vi "PH_VacuumControl.Show Trend.vi"(0 "i ref in":refnum<vi>, 5 "error in":errorcluster) -> (14 "i ref out":refnum<vi>, 19 "error out":errorcluster)   [LabVIEW 2014, in "PH_VacuumControl.lvlib"]
doc: "This VI shows the Trend data."
uses:
  PH_VacuumControl.lvlib
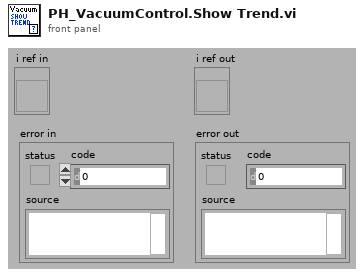
[diagram p1: front panel]
types:
  T1 = typedef "PH_VacuumControl.lvlib/PH_VacuumControl.i attribute.ctl" = cluster{"GUI Refs":cluster{"Exit":refnum<vi>, "Set Unit":refnum<vi>, "Device found":refnum<vi>, "Busy":refnum<vi>, "State":refnum<vi>, "Delete":refnum<vi>, "Channels":refnum<vi>, "Channel Name":refnum<vi>, "Trend":refnum<vi>, "Logarithmic":refnum<vi>, "Limit reached":refnum<vi>, "Channel Name 1 MT":refnum<vi>, "Channel Name 2 MT":refnum<vi>, "Trend MT":refnum<vi>, "Logarithmic MT":refnum<vi>, "Limit reached MT":refnum<vi>}, "Device found":bool, "Busy":bool, "Selected Unit":i32, "Channels [mbar]":T2, "Channel Names":cluster{"Channel 1":string, "Channel 2":string, "Channel 3":string, "Channel 4":string, "Channel 5":string, "Channel 6":string}, "Status":T3, "AGCxxx VISA Cluster":T4, "Instr Firmware Revision":string, "Service IDs Pressure":cluster{"Channel 1":i32, "Channel 2":i32, "Channel 3":i32, "Channel 4":i32, "Channel 5":i32, "Channel 6":i32}, "Service IDs Limits":cluster{"Channel 1":i32, "Channel 2":i32, "Channel 3":i32, "Channel 4":i32, "Channel 5":i32, "Channel 6":i32}, "Trend":cluster{"Start Point":timestamp, "Pressures [mbar] Channel 1":dbl[], "Pressures [mbar] Channel 2":dbl[], "Pressures [mbar] Channel 3":dbl[], "Pressures [mbar] Channel 4":dbl[], "Pressures [mbar] Channel 5":dbl[], "Pressures [mbar] Channel 6":dbl[], "Timebase [s]":i32[], "Trend Channel":u16, "Start Fit":dbl, "Trend Channel 1 MT":u16, "Trend Channel 2 MT":u16, "Start or continue Fit MT":dbl, "Continue or start Fit MT":dbl, "Datasets strored":i32, "Dataarray Size":i32}, "Running":bool}
  T2 = typedef "PH_VacuumControl.lvlib/PH_VacuumControl.Channels.ctl" = cluster{"Channel 1":dbl, "Channel 2":dbl, "Channel 3":dbl, "Channel 4":dbl, "Channel 5":dbl, "Channel 6":dbl, "Name Channel 1":string, "Name Channel 2":string, "Name Channel 3":string, "Name Channel 4":string, "Name Channel 5":string, "Name Channel 6":string, "Upper Limit":dbl, "Upper Limit 2":dbl, "Upper Limit 3":dbl, "Upper Limit 4":dbl, "Upper Limit 5":dbl, "Upper Limit 6":dbl}
  T3 = typedef "PH_StatusHandler.lvlib/PH_StatusHandler.Status.ctl" = i16
  T4 = typedef "AGCxxx - Driver.lvlib/AGCxxx VISA Control.ctl" = cluster{"VISA resource name":refnum<visa-resource-name>, "VISA Timeout Value (1000 ms)":u32, "Lock Timeout (1000 ms)":u32, "MAX Channel (6)":i32}
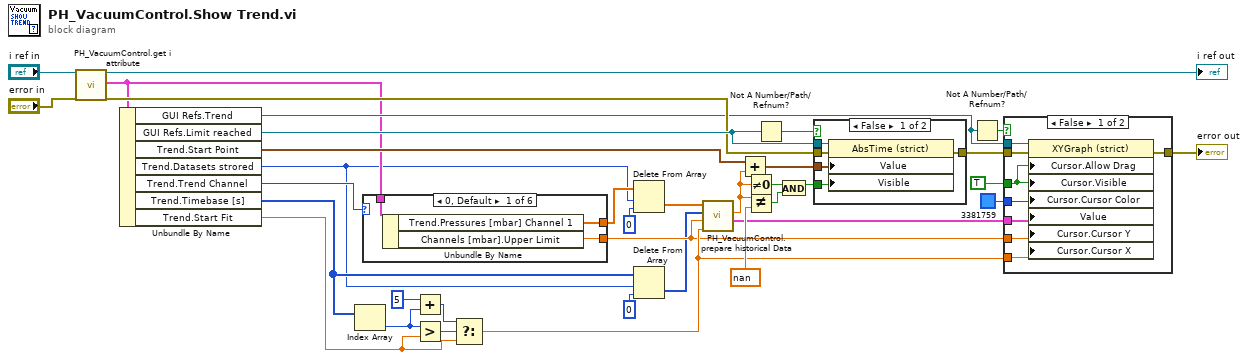
[diagram p0: block diagram]
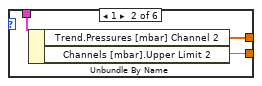
[diagram p4: hidden frame]
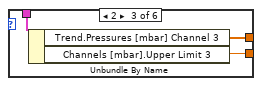
[diagram p5: hidden frame]
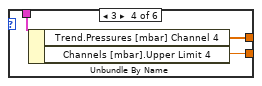
[diagram p6: hidden frame]
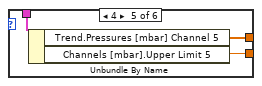
[diagram p7: hidden frame]
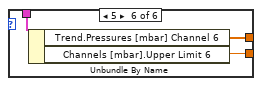
[diagram p8: hidden frame]
diagram:
  n1 = call "PH_VacuumControl.get i attribute.vi"("i ref in"="i ref in", "error in (no error)"="error in") -> ("i ref out"=→"i ref out":refnum<vi>, "i attribute"=w10:T1, "error out"=w27:errorcluster)  [unwired: 15 in]
  n2 = Unbundle By Name(w10) -> ("GUI Refs.Trend"=w23:refnum<vi>, "GUI Refs.Limit reached"=w29:refnum<vi>, "Trend.Start Point"=w31:timestamp, "Trend.Datasets strored"=w2:i32, "Trend.Trend Channel"=w11:u16, "Trend.Timebase [s]"=w16:i32[], "Trend.Start Fit"=w18:dbl)
  n3 = Index Array(array=w16) -> (element=w20:i32)  [unwired: 1 in]
  n4 = case shown="0, Default" w11 {
    tunnel: w10 -> [w39 w42 w45 w48 w51 w54]
    tunnel: [w38 w41 w44 w47 w50 w53] -> w3
    tunnel: [w37 w40 w43 w46 w49 w52] -> w15
    frame 0, Default {
      n5 = Unbundle By Name(w39) -> ("Trend.Pressures [mbar] Channel 1"=w38:dbl[], "Channels [mbar].Upper Limit"=w37:dbl)
    }
    frame 1 {
      n6 = Unbundle By Name(w42) -> ("Trend.Pressures [mbar] Channel 2"=w41:dbl[], "Channels [mbar].Upper Limit 2"=w40:dbl)
    }
    frame 2 {
      n7 = Unbundle By Name(w45) -> ("Trend.Pressures [mbar] Channel 3"=w44:dbl[], "Channels [mbar].Upper Limit 3"=w43:dbl)
    }
    frame 3 {
      n8 = Unbundle By Name(w48) -> ("Trend.Pressures [mbar] Channel 4"=w47:dbl[], "Channels [mbar].Upper Limit 4"=w46:dbl)
    }
    frame 4 {
      n9 = Unbundle By Name(w51) -> ("Trend.Pressures [mbar] Channel 5"=w50:dbl[], "Channels [mbar].Upper Limit 5"=w49:dbl)
    }
    frame 5 {
      n10 = Unbundle By Name(w54) -> ("Trend.Pressures [mbar] Channel 6"=w53:dbl[], "Channels [mbar].Upper Limit 6"=w52:dbl)
    }
  }
  n11 = Add(x=5, y=w20) -> (x+y=w22:i32)
  n12 = Greater?(x=w20, y=w18) -> (0:w17:bool)
  n13 = Select(t=w22, s=w17, f=w18) -> (s? t:f=w19:dbl)
  n14 = Delete From Array(array=w3, length=w2, index=0) -> (deleted portion=w4:dbl[])  [unwired: 1 out]
  n15 = Delete From Array(array=w16, length=w2, index=0) -> (deleted portion=w5:i32[])  [unwired: 1 out]
  n16 = call "PH_VacuumControl.prepare historical Data.vi"("Start Fit"=w19, "Limit"=w15, "Timebase [s]"=w5, "Pressure [mbar]"=w4) -> ("Trend"=w13:cluster{i32[], "Data":dbl[]}[], "Time to reach Limit"=w33:dbl)  [unwired: 5 in]
  n17 = Add(x=w31, y=w33) -> (x+y=w32:timestamp)
  n18 = Not Equal To 0?(x=w33) -> (x != 0?=w30:bool)
  n19 = Not Equal?(x=w33, y=nan) -> (x != y?=w36:bool)
  n20 = Not A Number/Path/Refnum?(number/path/refnum=w29) -> (NaN/Path/Refnum?=w26:bool)
  n21 = And(x=w30, y=w36) -> (x .and. y?=w35:bool)
  n22 = case shown="False" w26 {
    tunnel: w27 -> [w59 w60]
    tunnel: [w58 w60] -> w28
    tunnel: w29 -> [w57 _]
    tunnel: w32 -> [w56 _]
    tunnel: w35 -> [w55 _]
    frame False {
      n23 = property class="AbsTime (strict)"(reference=w57, error in=w59, "Value"=w56, "Visible"=w55) -> (error out=w58:errorcluster)  [unwired: 1 out]
    }
    frame True {
    }
  }
  n24 = Not A Number/Path/Refnum?(number/path/refnum=w23) -> (NaN/Path/Refnum?=w14:bool)
  n25 = case shown="False" w14 {
    tunnel: w28 -> [w68 w69]
    tunnel: [w67 w69] -> w12
    tunnel: w23 -> [w66 _]
    tunnel: w13 -> [w61 _]
    tunnel: w15 -> [w65 _]
    tunnel: w19 -> [w64 _]
    tunnel: TRUE ("Cursor.Allow Drag") -> [w63 _]
    tunnel: u32 3381759 ("Color Box") -> [w62 _]
    frame False {
      n26 = property class="XYGraph (strict)"(reference=w66, error in=w68, "Cursor.Allow Drag"=w63, "Cursor.Visible"=w63, "Cursor.Cursor Color"=w62, "Value"=w61, "Cursor.Cursor Y"=w65, "Cursor.Cursor X"=w64) -> (error out=w67:errorcluster)  [unwired: 1 out]
    }
    frame True {
    }
  }
  "error out" <- w12
